vi "Write WriteTimeout.vi"(8 "error in (no error)":errorcluster, 10 "WriteTimeout":i32=5000, 11 "TcpClient in":refnum<class "TcpClient.lvclass">) -> (0 "error out":errorcluster, 3 "TcpClient out":refnum<class "TcpClient.lvclass">)   [LabVIEW 2021, in "TcpClient.lvlib" / "TcpClient.lvclass"]
uses:
  TcpClient.lvclass
  TcpClient.lvclass/TcpClient.ctl
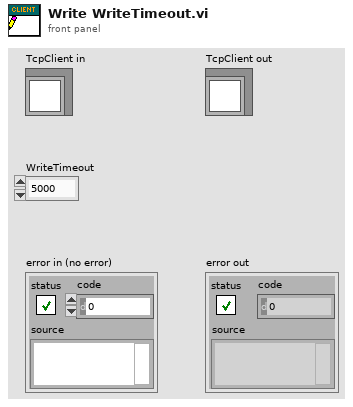
[diagram p1: front panel]
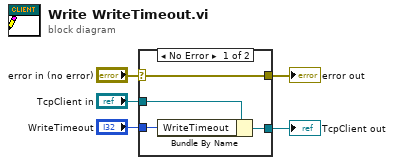
[diagram p0: block diagram]
diagram:
  n1 = case shown="No Error" "error in (no error)" {
    selector: "error in (no error)" -> [w9 w10]
    tunnel: [w9 w10] -> w4
    tunnel: [w7 w11] -> w2
    tunnel: "TcpClient in" -> [w8 w11]
    tunnel: "WriteTimeout" -> [w6 _]
    frame No Error {
      n2 = Bundle By Name(cluster=w8, "WriteTimeout"=w6) -> (w7:refnum<class "TcpClient.lvclass">)
    }
    frame Error {
    }
  }
  "error out" <- w4
  "TcpClient out" <- w2
